vi "Main-Nationa-remotel.vi"() -> ()   [LabVIEW 2019]
uses:
  <userlib>/KNR OS 4.0 LabVIEW Toolkit/F710/f710.ctl
  <vilib>/Platform/TimedLoop/XDataNode/timing_clust.ctl
  <vilib>/Platform/TimedLoop/XDataNode/nitl_modes.ctl
  <vilib>/Platform/TimedLoop/XDataNode/wakeup.ctl
  FPGA_subVIs/low level/motor/motor enum.ctl
  ctl/servo act.ctl
  ctl/remote.ctl
  ctl/height.ctl
  <vilib>/platform/TimedLoop/XDataNode/XDataNode.xnode
  <vilib>/Platform/TimedLoop/XDataNode/XDNodeRunTimeDep.lvlib
  FPGA_subVIs/low level/motor/motor.lvlib
  FPGA_subVIs/my FPGA lib.lvlib
panel:
  out "error out":errorcluster
  in  "stop":bool
  out "Numeric":dbl
  out "-x":dbl
  out "F710":T1
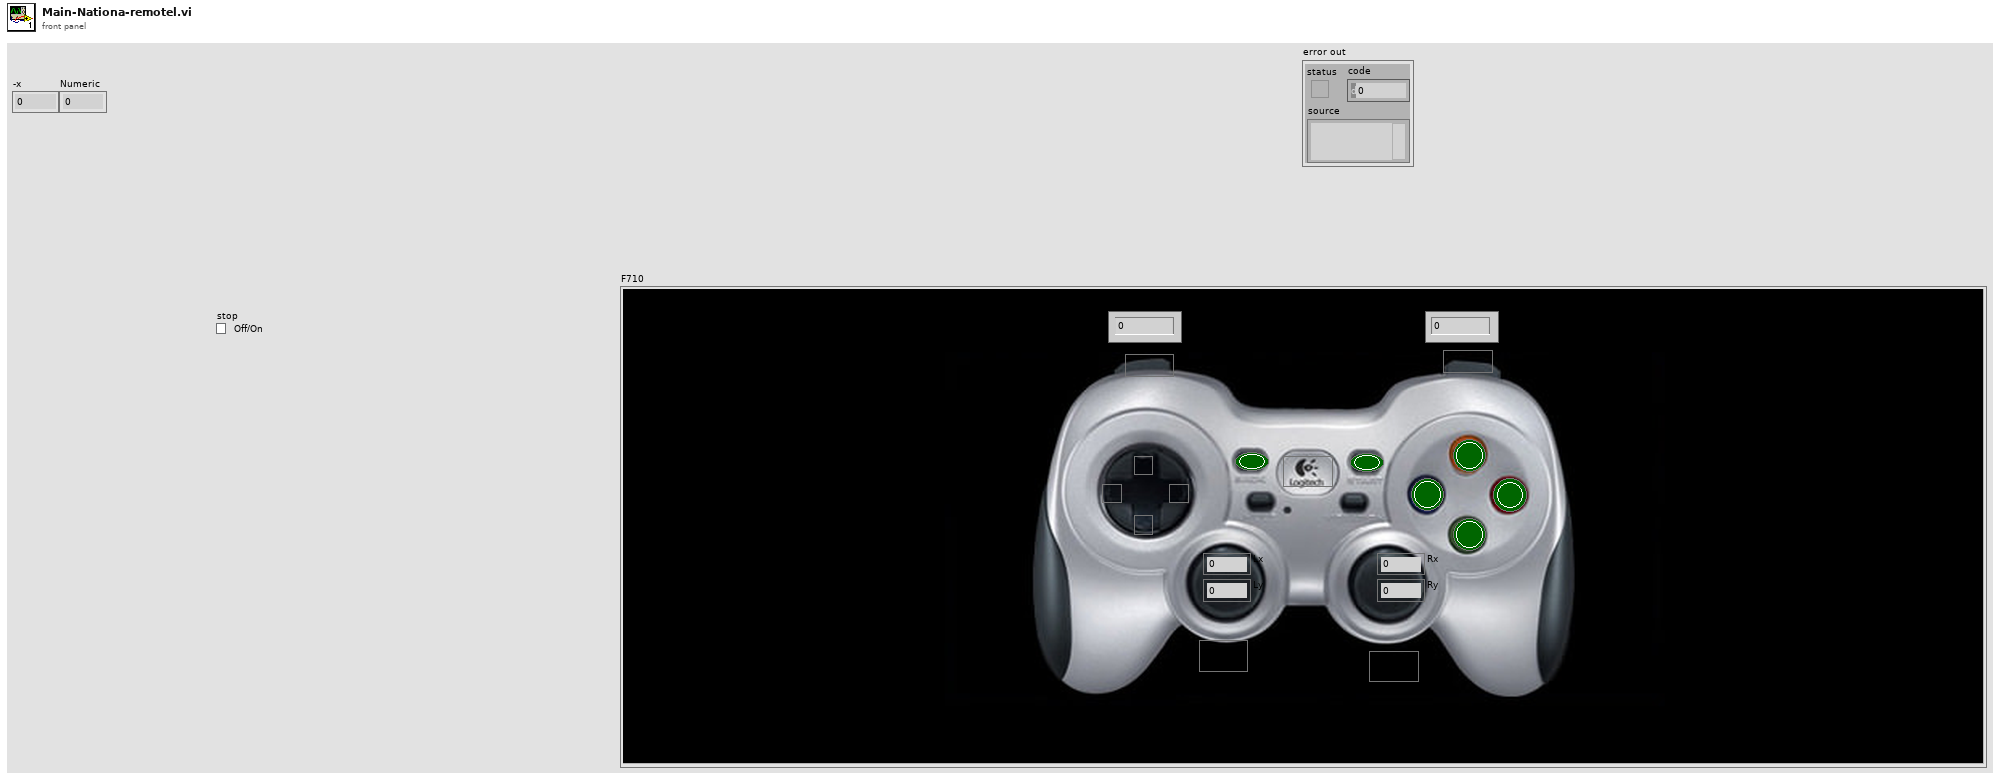
[diagram p1: front panel]
types:
  T1 = typedef "f710.ctl" = cluster{"Down":bool, "Left":bool, "Up":bool, "Right":bool, "A":bool, "X":bool, "Y":bool, "B":bool, "LB":bool, "RB":bool, "LT":i16, "RT":i16, "L3":bool, "R3":bool, "Ly":i16, "Lx":i16, "Ry":i16, "Rx":i16, "Back":bool, "Start":bool, "center":bool}
  T2 = typedef "XDNodeRunTimeDep.lvlib/timing_clust.ctl" = cluster{"Expected End [f-1]":u64, "Actual End [f-1]":u64, "Finished Late? [f-1]":bool, "Expected End [i-1]":u64, "Actual End [i-1]":u64, "Finished Late? [i-1]":bool, "Expected Start [i]":u64, "Actual Start [i]":u64, "Expected Start [f]":u64, "Actual Start [f]":u64, "Source Name":string, "Structure Name":string, "Period":i64, "Deadline":i64, "Offset":i64, "Start":i64, "Priority":i32, "Timeout":i32, "Mode":T3, "Wakeup Reason":T4, "Error":errorcluster, "Source Type":string, "Secondary Source Type":string, "Global End Time":u64, "Global Start Time":u64, "Frame Duration":u64, "Iteration Duration":u64, "Assigned CPU":i32, "I/O Scan Engine Mode":u32}
  T3 = typedef "XDNodeRunTimeDep.lvlib/nitl_modes.ctl" = enum32{"No Change", "Process missed periods, maintain original phase", "Discard missed periods, maintain original phase", "Process missed periods, ignore original phase", "Discard missed periods, ignore original phase"}
  T4 = typedef "XDNodeRunTimeDep.lvlib/wakeup.ctl" = enum32{"Normal", "Aborted", "Asynchronous wakeup", "Timing source error", "Timed loop error", "Timeout"}
  T5 = typedef "servo act.ctl" = enum16{"catch", "relax", "left idle", "center", "red relax", "left reg", "right reg"}
  T6 = cluster{"proportional gain (Kc)":dbl, "integral time (Ti, min)":dbl, "derivative time (Td, min)":dbl}
  T7 = typedef "my FPGA lib.lvlib/motor.lvlib/motor enum.ctl" = enum16{"M1", "M2", "M3", "M4"}
  T8 = typedef "remote.ctl" = cluster{"Motor speed":dbl[], "height":dbl, "dir":i32, "catch?":bool}
  T9 = typedef "height.ctl" = enum16{"IDLE", "recycle pre-catch", "recycle catch", "recycle zone", "vision height", "box 1", "box 2", "box 3", "box 1 pre", "box 2 pre", "box 3 pre", "reg 1", "reg 2", "reg 1 pre", "reg 2 pre", "put 1", "put 2", "put 3"}
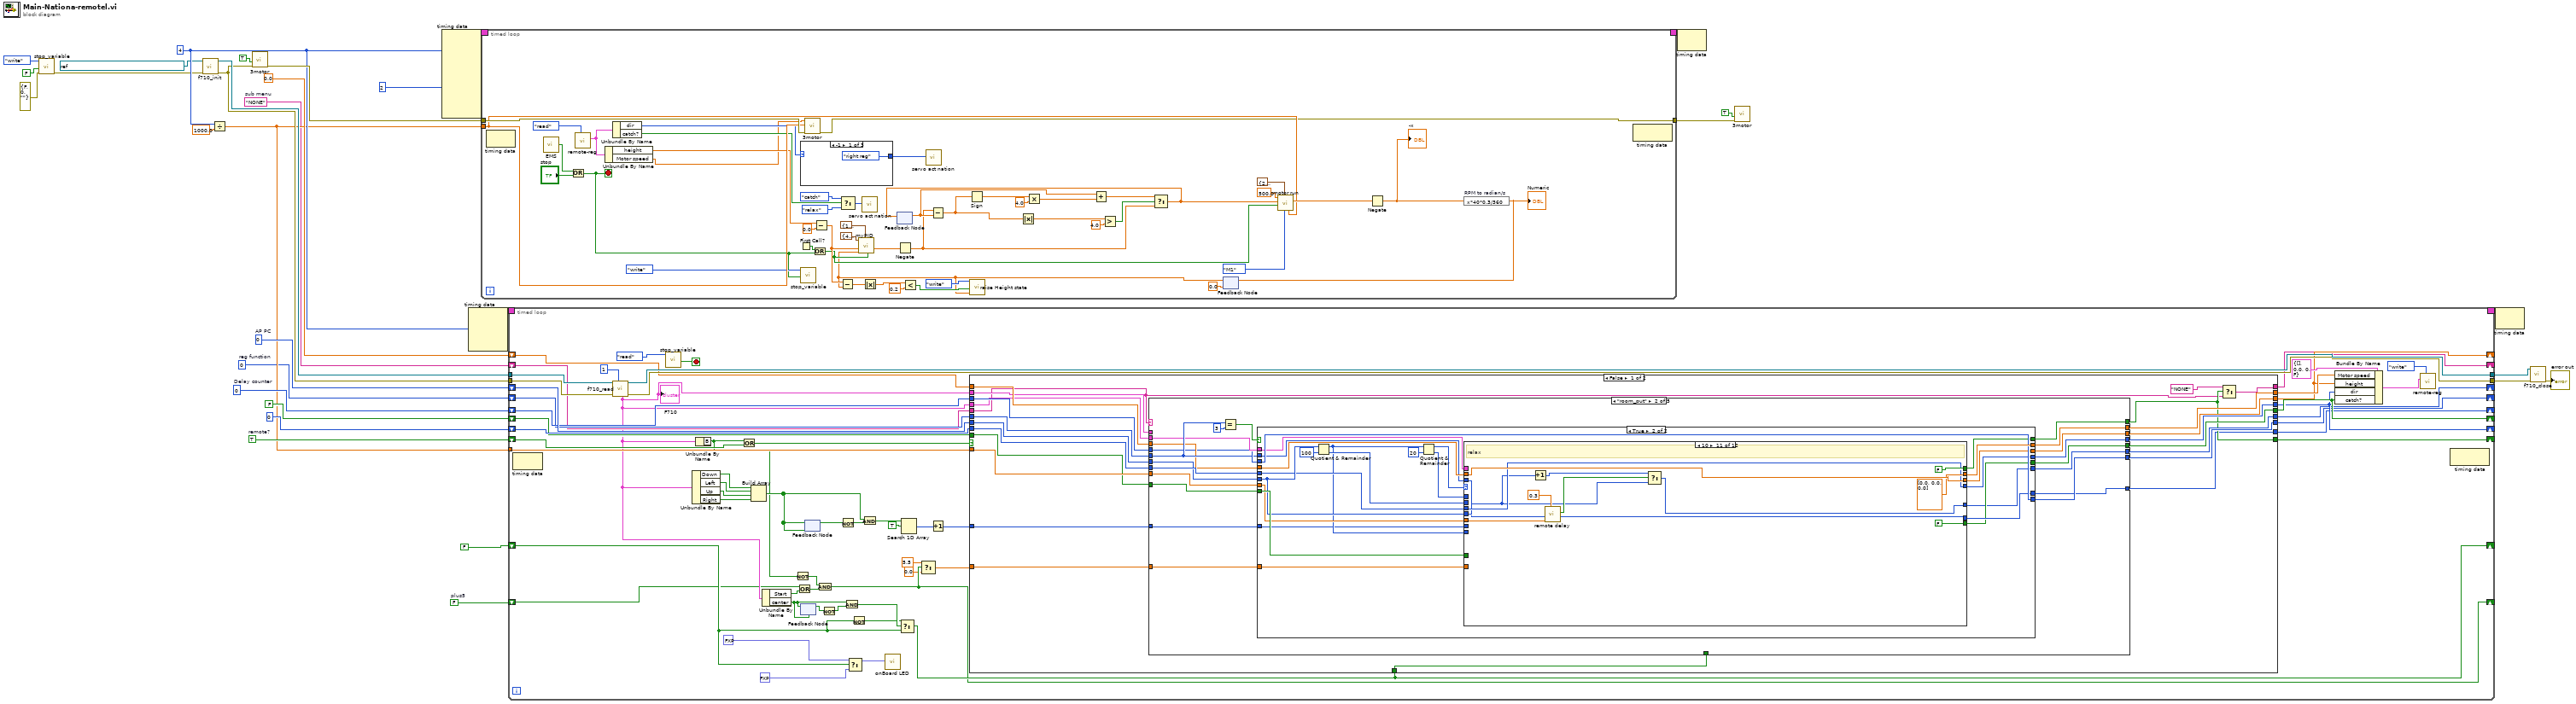
[diagram p0: block diagram]
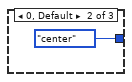
[diagram p2: hidden frame]
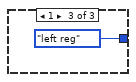
[diagram p3: hidden frame]
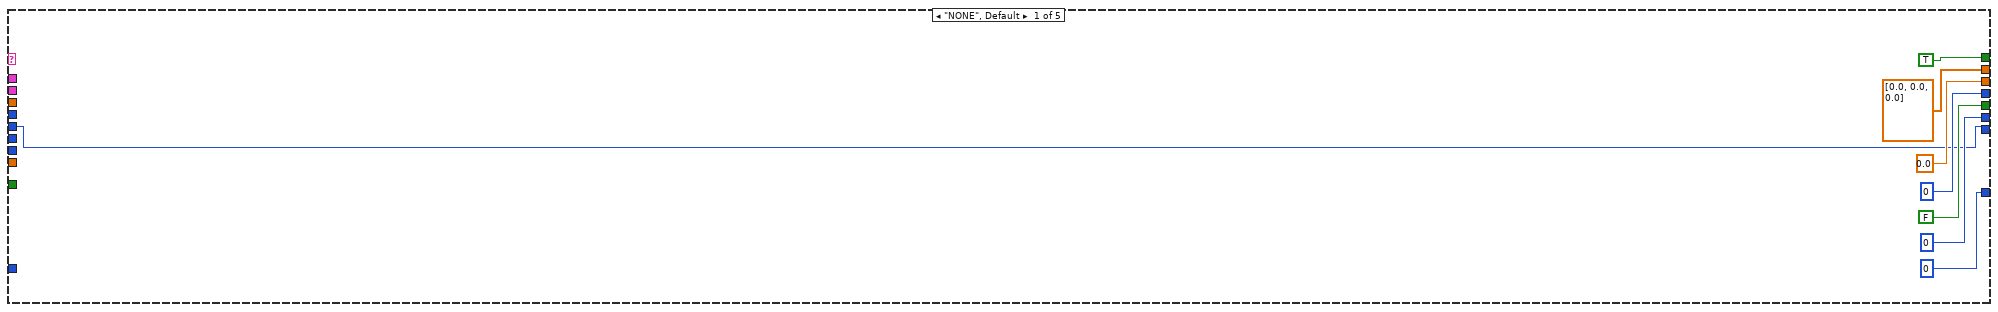
[diagram p4: hidden frame]
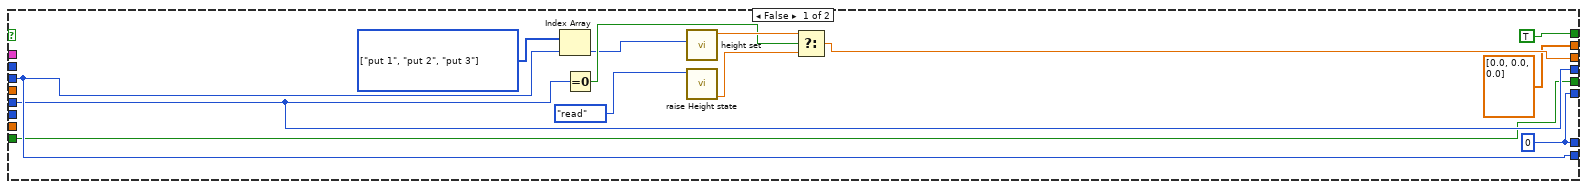
[diagram p5: hidden frame]
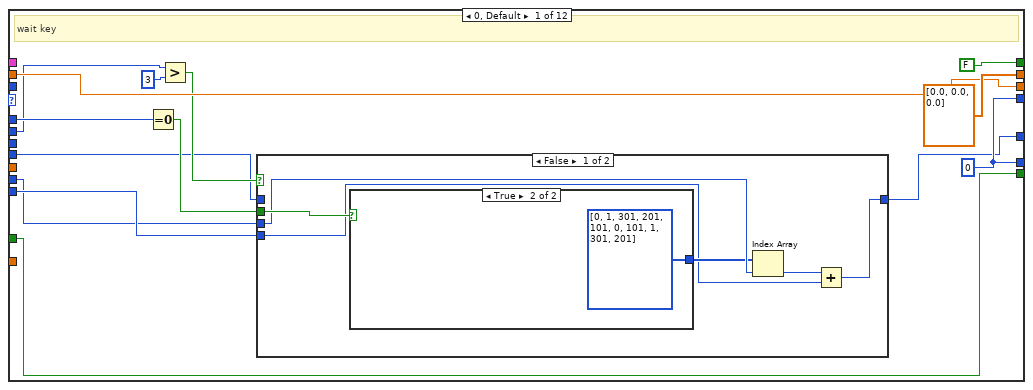
[diagram p6: hidden frame]
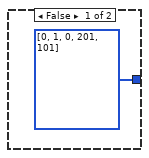
[diagram p7: hidden frame]
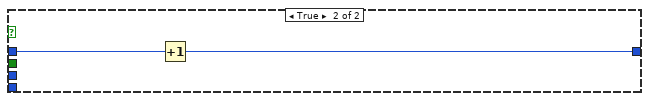
[diagram p8: hidden frame]
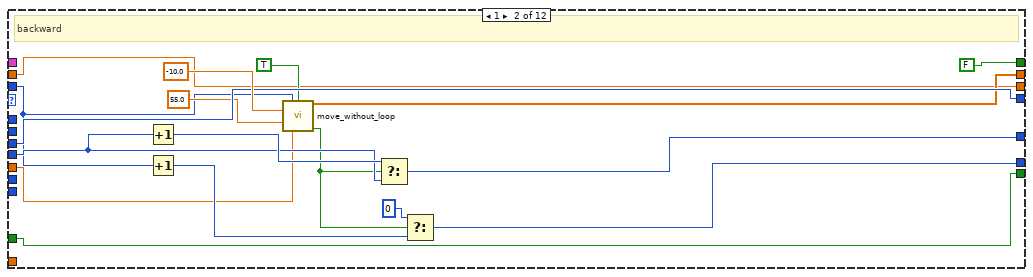
[diagram p9: hidden frame]
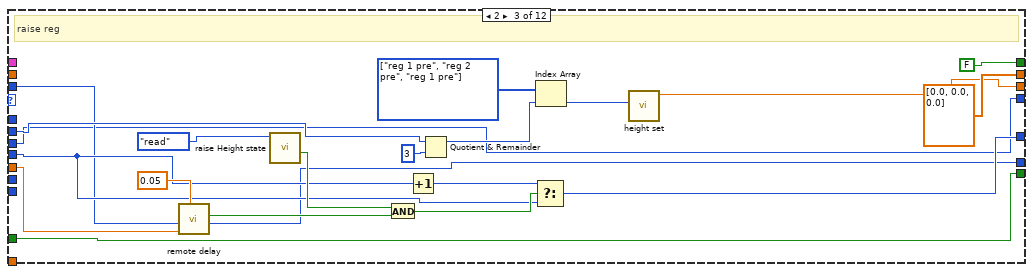
[diagram p10: hidden frame]
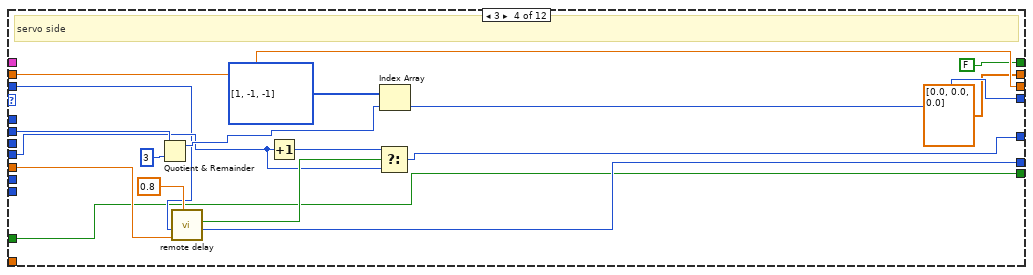
[diagram p11: hidden frame]
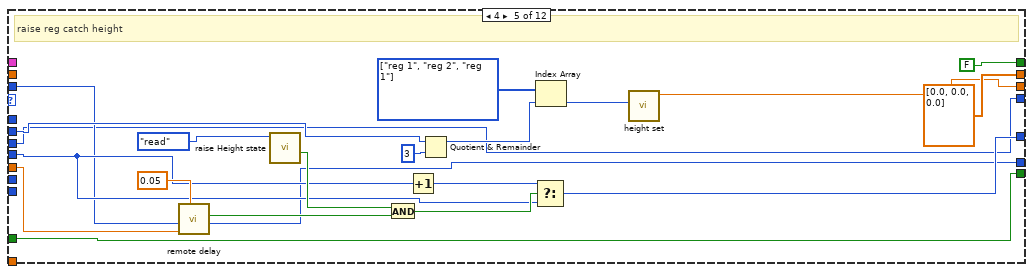
[diagram p12: hidden frame]
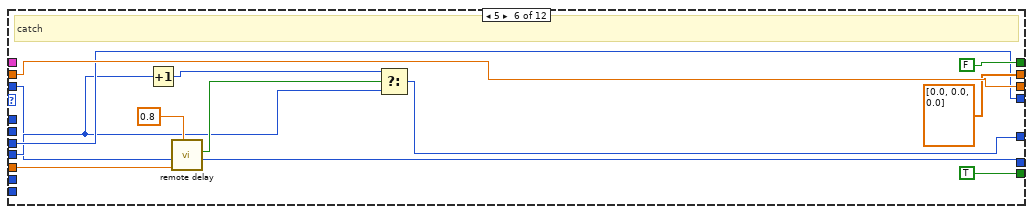
[diagram p13: hidden frame]
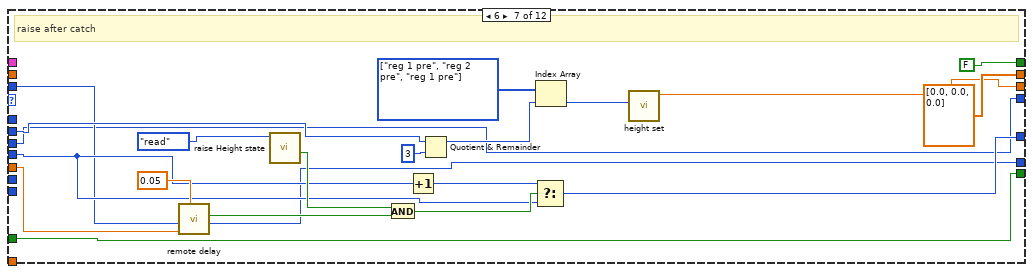
[diagram p14: hidden frame]
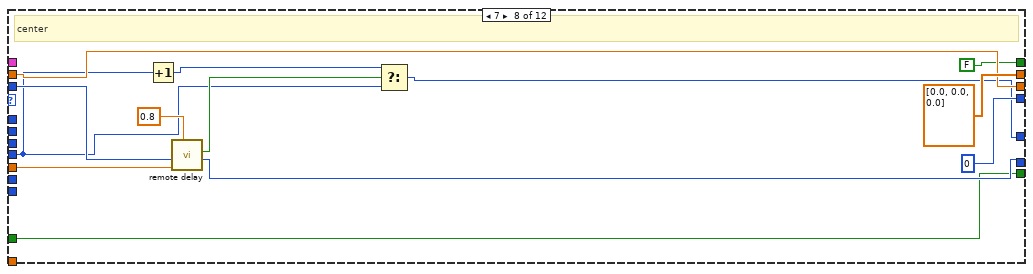
[diagram p15: hidden frame]
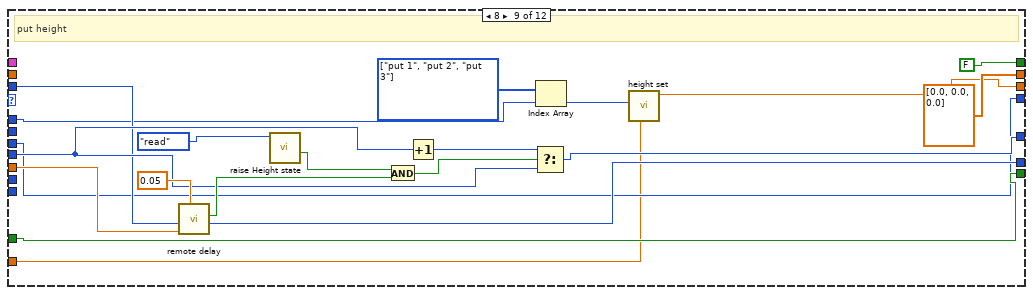
[diagram p16: hidden frame]
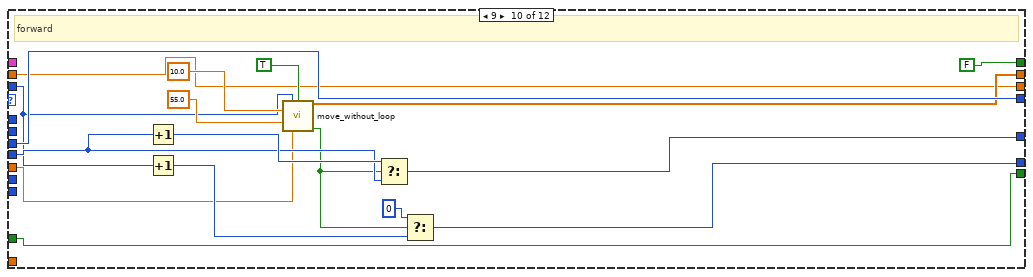
[diagram p17: hidden frame]
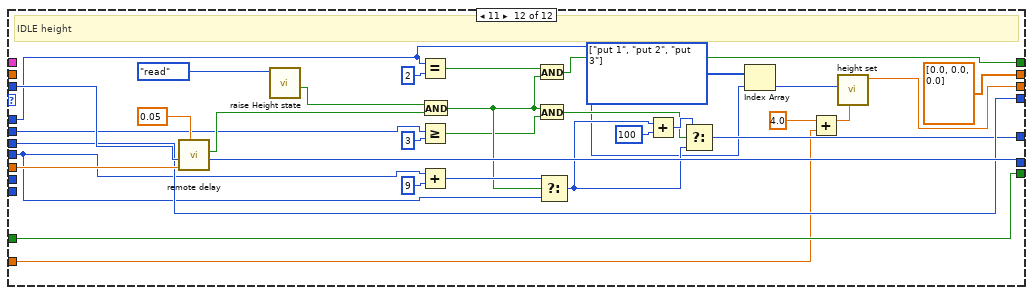
[diagram p18: hidden frame]
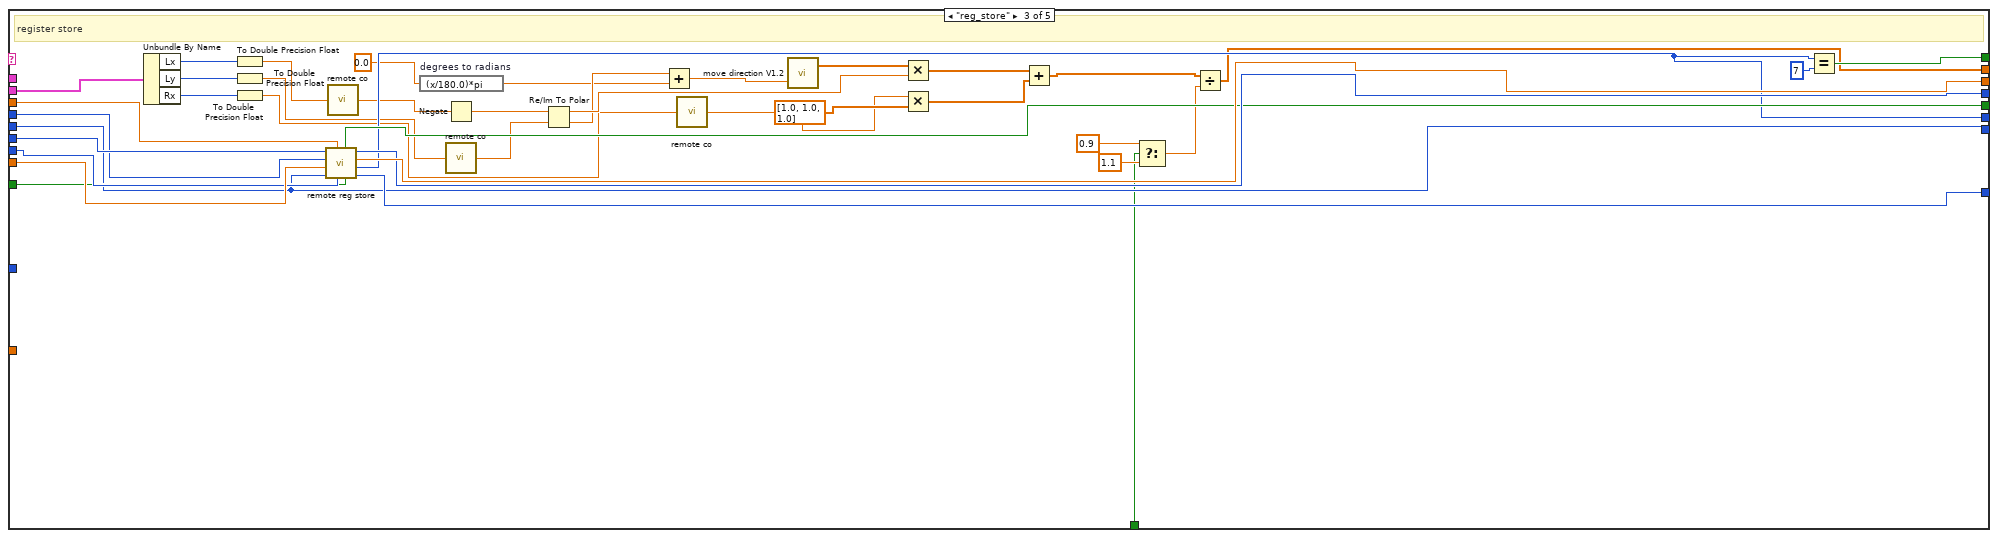
[diagram p19: hidden frame]
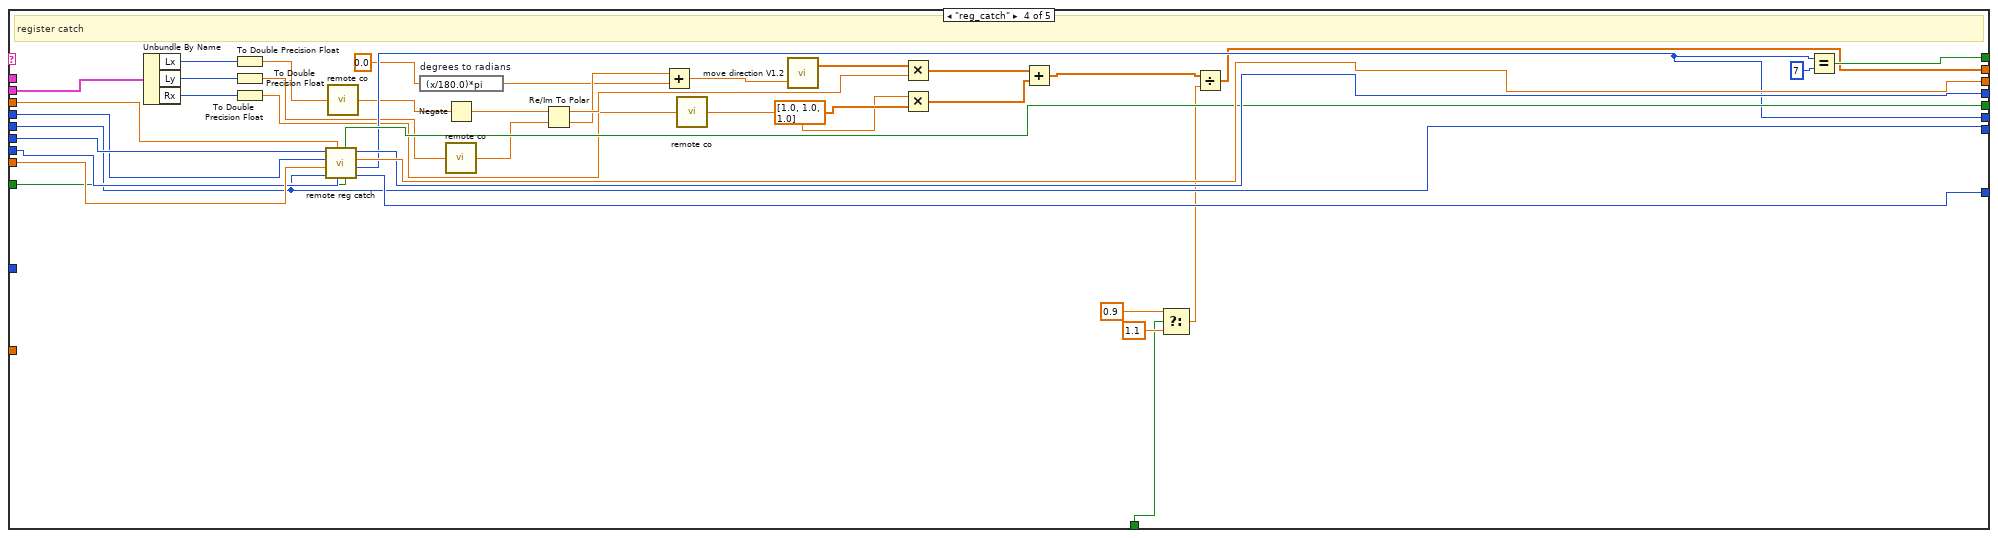
[diagram p20: hidden frame]
diagram:
  w1 = FALSE  # plus5
  w3 = "NONE"  # sub menu
  w4 = 0  # reg function
  w6 = 0  # Delay counter
  w7 = 0  # AP PC
  w8 = TRUE  # remote?
  w23 = i64 4 ("Period")
  n1 = call "stop_variable.vi"("Error In"=errorcluster {"status"=FALSE, "code"=0, "source"=""} ("error in (no error)"), "Write"=FALSE, "Enum"=enum16{"read", "write"}."write") -> ("Error Out"=w12:errorcluster)  [unwired: 7 in, 1 out]
  n2 = call <userlib>:"f710_init.vi"("error in (no error)"=w12, "USB RAW VISA resource name"=refnum<visa-resource-name> "USB0::0x046D::0xC21F::EEAB948F::RAW") -> ("error out"=w11:errorcluster, "VISA Refnum out"=w30:refnum<visa-resource-name>)  [unwired: 8 in]
  n3 = Divide(x=w23, y=1000.0) -> (x/y=w5:dbl)
  n4 = call "3motor.vi"("error in (no error)"=w11, "Reset"=TRUE) -> ("error out"=w25:errorcluster)  [unwired: 8 in, 1 out]
  n5 = node-c288(w23, i64 2 ("Offset")) -> (w27:T2)  [unwired: 8 in]
  n6 = node-c288(w23) -> (w32:T2)  [unwired: 3 in]
  n7 = timed-loop {
    timing: w27 -> [_]
    timing-out: [_] -> w26
    tunnel: w25 -> [w80]
    tunnel: w5 -> [w46]
    tunnel: [w36] -> w21
    stop <- w34 stop-if-true
    n8 = node-c288() -> ()  [unwired: 1 in, 1 out]
    n9 = call "EMS.vi"() -> ("A/DIO4 (Pin 19)"=w61:bool)
    n10 = Or(x=w61, y="stop") -> (x .or. y?=w34:bool)
    n11 = call "remote-reg.vi"("Enum"=enum16{"read", "write"}."read") -> ("read"=w43:T8)  [unwired: 10 in]
    n12 = Unbundle By Name(w43) -> ("height"=w44:dbl, "Motor speed"=w33:dbl[])
    n13 = Unbundle By Name(w43) -> ("dir"=w38:i32, "catch?"=w42:bool)
    n14 = First Call?() -> (First Call?: T/F=w51:bool)
    n15 = case shown="-1" w38 {
      tunnel: [servo_act."right reg" ("servo act") servo_act."center" ("servo act") servo_act."left reg" ("servo act")] -> w37
      frame -1 {
      }
      frame 0, Default {
      }
      frame 1 {
      }
    }
    n16 = call "stop_variable.vi"("Write"=w34, "Enum"=enum16{"read", "write"}."write") -> ()  [unwired: 8 in, 2 out]
    n17 = call "3motor.vi"("error in (no error)"=w80, "dt(s)"=w46, "Motor speed"=w33) -> ("error out"=w36:errorcluster)  [unwired: 7 in, 1 out]
    n18 = Or(x=w51, y=w34) -> (x .or. y?=w48:bool)
    n19 = Subtract(x=w44, y=0.0 ("x")) -> (x-y=w60:dbl)
    n20 = Select(t=servo_act."catch" ("servo act"), s=w42, f=servo_act."relax" ("servo act")) -> (s? t:f=w39:T5)
    n21 = call "servo act nation.vi"("servo act"=w39) -> ()  [unwired: 10 in, 1 out]
    n22 = feedback #1() -> (w71:dbl)  [unwired: 1 in]
    n23 = call "servo act nation.vi"("servo act"=w37) -> ()  [unwired: 10 in, 1 out]
    n24 = feedback #2(0.0) -> (w47:dbl)
    n25 = Subtract(x=w60, y=w47) -> (x-y=w59:dbl)
    n26 = call "myPID.vi"("s"=w48, "output range"=cluster{"output high":dbl, "output low":dbl} {"output high"=140.0, "output low"=-140.0}, "Processer"=w47, "setpoint"=w60, "PID"=cluster{"Kp":dbl, "Ki":dbl, "Kd":dbl} {"Kp"=45.0, "Ki"=0.0, "Kd"=0.0002}) -> ("out"=w75:dbl)  [unwired: 5 in, 1 out]
    n27 = Absolute Value(x=w59) -> (abs(x)=w58:dbl)
    n28 = Negate(x=w75) -> (-x=w66:dbl)
    n29 = Less?(x=w58, y=0.2) -> (x < y?=w56:bool)
    n30 = Subtract(x=w66, y=w71) -> (x-y=w65:dbl)
    n31 = Sign(1:w65) -> (0:w70:dbl)
    n32 = call "raise Height state.vi"("Write Height"=w47, "Write"=w56, "Enum"=enum16{"read", "write"}."write") -> ()  [unwired: 7 in, 2 out]
    n33 = Absolute Value(x=w65) -> (abs(x)=w74:dbl)
    n34 = Multiply(x=w70, y=4.0) -> (x*y=w68:dbl)
    n35 = Add(x=w71, y=w68) -> (x+y=w67:dbl)
    n36 = Greater?(x=w74, y=4.0) -> (0:w72:bool)
    n37 = Select(t=w67, s=w72, f=w66) -> (s? t:f=w53:dbl)
    n38 = feedback-in #1(w53) -> ()
    n39 = call "motor run.vi"("dt(s)"=w46, "motor select"=motor_enum."M1", "PID gains"=T6 {"proportional gain (Kc)"=20.0, "integral time (Ti, min)"=0.0, "derivative time (Td, min)"=0.0002}, "Reset"=w48, "speed RPM"=w53, "PWM frequence"=500.0) -> ("encoder"=w49:dbl)  [unwired: 2 in, 3 out]
    n40 = Negate(x=w49) -> (-x=w76:dbl)
    "-x" <- w76
    n41 = expression code="x*40*0.3/360" "RPM to radian/s"(w76) -> (w63:dbl)
    "Numeric" <- w63
    n42 = feedback-in #2(w63) -> ()
    n43 = node-c288() -> ()  [unwired: 1 in, 1 out]
  }
  n44 = timed-loop {
    timing: w32 -> [_]
    timing-out: [_] -> w31
    tunnel: w11 -> [w145]
    tunnel: w30 -> [w144]
    tunnel: [w143] -> w29
    tunnel: [w142] -> w28
    shift-right: [w129] -> _
    shift-left: 0.0 -> [w136]
    shift-right: [w128] -> _
    shift-left: 0 -> [w133]
    shift-right: [w130] -> _
    shift-left: FALSE -> [w132]
    shift-right: [w127] -> _
    shift-left: w8 -> [w131]
    shift-right: [w125] -> _
    shift-left: w7 -> [w126]
    shift-right: [w123] -> _
    shift-left: w6 -> [w124]
    tunnel: w5 -> [w122]
    shift-right: [w120] -> _
    shift-left: w4 -> [w121]
    shift-right: [w117] -> _
    shift-left: w3 -> [w118]
    shift-right: [w99] -> _
    shift-left: FALSE -> [w96]
    shift-right: [w89] -> _
    shift-left: w1 -> [w94]
    stop <- w140 stop-if-true
    n45 = node-c288() -> ()  [unwired: 1 in, 1 out]
    n46 = call <userlib>:"f710_read.vi"("Timeout to wait for Interrupt (ms)"=u32 1, "error in (no error)"=w145, "VISA Refnum in"=w144) -> ("error out"=w142:errorcluster, "VISA Refnum out"=w143:refnum<visa-resource-name>, "F710"=w102:T1)  [unwired: 6 in]
    "F710" <- w102
    n47 = call "stop_variable.vi"("Enum"=enum16{"read", "write"}."read") -> ("read"=w140:bool)  [unwired: 9 in, 1 out]
    n48 = Unbundle By Name(w102) -> ("Down"=w112:bool, "Left"=w113:bool, "Up"=w114:bool, "Right"=w115:bool)
    n49 = Unbundle By Name(w102) -> ("B"=w90:bool)
    n50 = Or(x=w90, y=w131) -> (x .or. y?=w119:bool)
    n51 = Build Array(w112, w113, w114, w115) -> (w109:bool[])
    n52 = Unbundle By Name(w102) -> ("Start"=w93:bool, "center"=w105:bool)
    n53 = Not(x=w90) -> (.not. x?=w91:bool)
    n54 = Or(x=w94, y=w93) -> (x .or. y?=w92:bool)
    n55 = feedback #3(w105) -> (w103:bool)
    n56 = feedback-in #3(w105) -> ()
    n57 = feedback #4(w109) -> (w108:bool[])
    n58 = feedback-in #4(w109) -> ()
    n59 = And(x=w91, y=w92) -> (x .and. y?=w89:bool)
    n60 = Not(x=w103) -> (.not. x?=w104:bool)
    n61 = Not(x=w108) -> (.not. x?=w110:bool[])
    n62 = And(x=w105, y=w104) -> (x .and. y?=w101:bool)
    n63 = Select(t=fxp<+,4,4> 15.0 ("OnBoard.LED[3:0]"), s=w96, f=fxp<+,4,4> 0.0 ("OnBoard.LED[3:0]")) -> (s? t:f=w97:fxp<+,4,4>)
    n64 = Not(x=w96) -> (.not. x?=w100:bool)
    n65 = And(x=w109, y=w110) -> (x .and. y?=w111:bool[])
    n66 = call "onBoard LED.vi"("OnBoard.LED[3:0]"=w97) -> ()  [unwired: 10 in, 1 out]
    n67 = Select(t=w100, s=w101, f=w96) -> (s? t:f=w99:bool)
    n68 = Search 1D Array(1D array=w111, element=TRUE) -> (index of element=w116:i32)  [unwired: 1 in]
    n69 = Select(t=5.5, s=w89, f=0.0) -> (s? t:f=w86:dbl)
    n70 = Increment(x=w116) -> (x+1=w106:i32)
    n71 = case shown="False" w119 {
      selector: w119 -> [_ w591]
      tunnel: [w168 w630] -> w137
      tunnel: w136 -> [w164 w623]
      tunnel: [w165 w569] -> w129
      tunnel: w102 -> [w157 w559]
      tunnel: w133 -> [w160 w613]
      tunnel: [w162 w593] -> w128
      tunnel: w132 -> [w159 w596]
      tunnel: [w158 w595] -> w130
      tunnel: [w153 w592] -> w127
      tunnel: w126 -> [w167 _]
      tunnel: [w163 w589] -> w125
      tunnel: w124 -> [w166 _]
      tunnel: [w149 w589] -> w123
      tunnel: w122 -> [w161 _]
      tunnel: w102 -> [w156 _]
      tunnel: w121 -> [w155 _]
      tunnel: [w154 w574] -> w120
      tunnel: w118 -> [w152 w571]
      tunnel: [w150 w576] -> w117
      tunnel: w106 -> [w148 _]
      tunnel: w99 -> [w147 w557]
      tunnel: w86 -> [w146 _]
      frame False {
        n72 = case shown="\"room_put\"" w152 {
          tunnel: [dbl[] [0.0, 0.0, 0.0] w184 w466 w506 dbl[] [0.0, 0.0, 0.0]] -> w168
          tunnel: w167 -> [_ w183 w501 w541 _]
          tunnel: w166 -> [_ w180 w500 w540 _]
          tunnel: [0.0 ("upper limit") w190 w499 w539 w546] -> w165
          tunnel: w164 -> [_ w182 w498 w538 _]
          tunnel: [0 ("Delay counter") w187 w497 w537 0 ("delay timer out")] -> w149
          tunnel: [0 w188 w490 w530 0 ("PC out")] -> w163
          tunnel: [0 w191 w496 w536 w550] -> w162
          tunnel: w161 -> [_ w179 w495 w535 _]
          tunnel: w160 -> [_ w192 w494 w534 w550]
          tunnel: w159 -> [_ w185 w493 w533 w553]
          tunnel: [FALSE w186 w492 w532 w553] -> w158
          tunnel: [TRUE w189 w491 w531 TRUE] -> w153
          tunnel: w157 -> [_ w181 w467 w507 _]
          tunnel: w156 -> [_ _ _ _ _]
          tunnel: w155 -> [w169 w194 w488 w528 w542]
          tunnel: [w169 w193 w488 w528 w542] -> w154
          tunnel: w148 -> [_ w178 _ _ _]
          tunnel: w147 -> [_ _ w462 w503 _]
          tunnel: w146 -> [_ w177 _ _ _]
          frame "NONE", Default {
          }
          frame "room_put" {
            n73 = Equal?(x=w194, y=3) -> (x = y?=w195:bool)
            n74 = case shown="True" w195 {
              tunnel: w194 -> [w203 w231]
              tunnel: [w203 w231] -> w193
              tunnel: w192 -> [w202 w215]
              tunnel: [w202 w230] -> w191
              tunnel: [w201 w225] -> w190
              tunnel: [TRUE w228] -> w189
              tunnel: [w199 w216] -> w188
              tunnel: [w199 w229] -> w187
              tunnel: [w198 w227] -> w186
              tunnel: w185 -> [w198 w226]
              tunnel: [dbl[] [0.0, 0.0, 0.0] w232] -> w184
              tunnel: w183 -> [_ w217]
              tunnel: w182 -> [_ w224]
              tunnel: w181 -> [_ w223]
              tunnel: w180 -> [_ w214]
              tunnel: w179 -> [_ w213]
              tunnel: w178 -> [_ w211]
              tunnel: w177 -> [_ w210]
              frame False {
                w199 = 0
                w205 = T9[] [enum."put 1", enum."put 2", enum."put 3"] items=["IDLE", "recycle pre-catch", "recycle catch", "recycle zone", "vision height", "box 1", "box 2", "box 3", "box 1 pre", "box 2 pre", "box 3 pre", "reg 1", "reg 2", "reg 1 pre", "reg 2 pre", "put 1", "put 2", "put 3"] ("height name")
                n75 = Index Array(array=w205, index=w203) -> (element=w204:T9)
                n76 = Equal To 0?(x=w202) -> (x = 0?=w208:bool)
                n77 = call "height set.vi"("height name"=w204) -> ("Numeric"=w209:dbl)  [unwired: 10 in]
                n78 = call "raise Height state.vi"("Enum"=enum16{"read", "write"}."read") -> ("read Height"=w206:dbl)  [unwired: 9 in, 1 out]
                n79 = Select(t=w209, s=w208, f=w206) -> (s? t:f=w201:dbl)
              }
              frame True {
                n80 = Quotient & Remainder(x=w217, y=100) -> (x-y*floor(x/y)=w212:i32, floor(x/y)=w218:i32)
                n81 = Quotient & Remainder(x=w212, y=20) -> (x-y*floor(x/y)=w221:i32, floor(x/y)=w220:i32)
                n82 = case shown="10" w221 {
                  tunnel: [dbl[] [0.0, 0.0, 0.0] w260 dbl[] [0.0, 0.0, 0.0] dbl[] [0.0, 0.0, 0.0] dbl[] [0.0, 0.0, 0.0] dbl[] [0.0, 0.0, 0.0] dbl[] [0.0, 0.0, 0.0] dbl[] [0.0, 0.0, 0.0] dbl[] [0.0, 0.0, 0.0] w403 dbl[] [0.0, 0.0, 0.0] dbl[] [0.0, 0.0, 0.0]] -> w232
                  tunnel: [w245 w272 w274 w307 w312 w341 w346 0 ("Numeric") w382 w415 w425 w452] -> w230
                  tunnel: [w245 w267 w278 w298 w316 w336 w350 w373 w386 w410 w420 w456] -> w229
                  tunnel: [FALSE FALSE FALSE FALSE FALSE FALSE FALSE FALSE FALSE FALSE FALSE w446] -> w228
                  tunnel: [w243 w258 w275 w295 w313 TRUE w347 w367 w383 w401 FALSE w453] -> w227
                  tunnel: w226 -> [w243 w258 w275 w295 w313 _ w347 w367 w383 w401 _ w453]
                  tunnel: [w242 w257 w288 w306 w326 w343 w360 w377 w396 w400 w427 w434] -> w225
                  tunnel: w224 -> [w242 w257 _ w306 _ w343 _ w377 _ w400 w427 _]
                  tunnel: w223 -> [_ _ _ _ _ _ _ _ _ _ _ _]
                  tunnel: w220 -> [w241 _ _ _ _ _ _ _ w381 _ _ w432]
                  tunnel: w218 -> [w239 _ w294 w310 w332 _ w366 _ _ _ _ w444]
                  tunnel: w217 -> [w236 w269 w279 w299 w317 w337 w351 w370 w387 w412 w421 w450]
                  tunnel: [w235 w271 w280 w300 w318 w335 w352 w369 w388 w414 w419 w445] -> w216
                  tunnel: w215 -> [_ w272 w274 _ w312 w341 w346 _ w382 w415 w425 w452]
                  tunnel: w214 -> [_ w262 w277 w297 w315 w334 w349 w372 w385 w405 w418 w455]
                  tunnel: w213 -> [_ w264 w276 w296 w314 w333 w348 w371 w384 w407 w417 w454]
                  tunnel: w212 -> [w234 _ _ _ _ _ _ _ _ _ _ _]
                  tunnel: w211 -> [w233 _ _ _ _ _ _ _ _ _ _ _]
                  tunnel: w210 -> [_ _ _ _ _ _ _ _ w380 _ _ w430]
                  frame 0, Default {
                    w245 = 0
                    # "wait key"
                    n83 = Equal To 0?(x=w241) -> (x = 0?=w240:bool)
                    n84 = Greater?(x=w239, y=3) -> (0:w237:bool)
                    n85 = case shown="False" w237 {
                      tunnel: w240 -> [w252 _]
                      tunnel: w233 -> [w251 _]
                      tunnel: w236 -> [_ w256]
                      tunnel: [w248 w255] -> w235
                      tunnel: w234 -> [w247 _]
                      frame False {
                        n86 = case shown="True" w252 {
                          tunnel: [i32[] [0, 1, 0, 201, 101] i32[] [0, 1, 301, 201, 101, 0, 101, 1, 301, 201]] -> w250
                          frame False {
                          }
                          frame True {
                          }
                        }
                        n87 = Index Array(array=w250, index=w251) -> (element=w249:i32)
                        n88 = Add(x=w249, y=w247) -> (x+y=w248:i32)
                      }
                      frame True {
                        n89 = Increment(x=w256) -> (x+1=w255:i32)
                      }
                    }
                  }
                  frame 1 {
                    # "backward"
                    n90 = Increment(x=w269) -> (x+1=w270:i32)
                    n91 = Increment(x=w262) -> (x+1=w268:i32)
                    n92 = call "move_without_loop.vi"("i"=w262, "run"=TRUE, "Y"=-10.0, "speed"=55.0, "dt"=w264) -> ("speed out"=w260:dbl[], "complet"=w266:bool)  [unwired: 6 in, 3 out]
                    n93 = Select(t=w270, s=w266, f=w269) -> (s? t:f=w271:i32)
                    n94 = Select(t=0, s=w266, f=w268) -> (s? t:f=w267:i32)
                  }
                  frame 2 {
                    w292 = T9[] [enum."reg 1 pre", enum."reg 2 pre", enum."reg 1 pre"] items=["IDLE", "recycle pre-catch", "recycle catch", "recycle zone", "vision height", "box 1", "box 2", "box 3", "box 1 pre", "box 2 pre", "box 3 pre", "reg 1", "reg 2", "reg 1 pre", "reg 2 pre", "put 1", "put 2", "put 3"] ("height name")
                    # "raise reg"
                    n95 = call "remote delay.vi"("second"=0.05, "dt(s)"=w276, "i"=w277) -> ("i out"=w278:i32, "finish?"=w282:bool)  [unwired: 7 in]
                    n96 = call "raise Height state.vi"("Enum"=enum16{"read", "write"}."read") -> ("read"=w283:bool)  [unwired: 9 in, 1 out]
                    n97 = And(x=w283, y=w282) -> (x .and. y?=w281:bool)
                    n98 = Increment(x=w279) -> (x+1=w285:i32)
                    n99 = Quotient & Remainder(x=w294, y=3) -> (x-y*floor(x/y)=w289:i32)  [unwired: 1 out]
                    n100 = Select(t=w285, s=w281, f=w279) -> (s? t:f=w280:i32)
                    n101 = Index Array(array=w292, index=w289) -> (element=w291:T9)
                    n102 = call "height set.vi"("height name"=w291) -> ("Numeric"=w288:dbl)  [unwired: 10 in]
                  }
                  frame 3 {
                    # "servo side"
                    n103 = Quotient & Remainder(x=w310, y=3) -> (x-y*floor(x/y)=w308:i32)  [unwired: 1 out]
                    n104 = call "remote delay.vi"("second"=0.8, "dt(s)"=w296, "i"=w297) -> ("i out"=w298:i32, "finish?"=w302:bool)  [unwired: 7 in]
                    n105 = Increment(x=w299) -> (x+1=w301:i32)
                    n106 = Select(t=w301, s=w302, f=w299) -> (s? t:f=w300:i32)
                    n107 = Index Array(array=i32[] [1, -1, -1], index=w308) -> (element=w307:i32)
                  }
                  frame 4 {
                    w330 = T9[] [enum."reg 1", enum."reg 2", enum."reg 1"] items=["IDLE", "recycle pre-catch", "recycle catch", "recycle zone", "vision height", "box 1", "box 2", "box 3", "box 1 pre", "box 2 pre", "box 3 pre", "reg 1", "reg 2", "reg 1 pre", "reg 2 pre", "put 1", "put 2", "put 3"] ("height name")
                    # "raise reg catch height"
                    n108 = call "remote delay.vi"("second"=0.05, "dt(s)"=w314, "i"=w315) -> ("i out"=w316:i32, "finish?"=w320:bool)  [unwired: 7 in]
                    n109 = call "raise Height state.vi"("Enum"=enum16{"read", "write"}."read") -> ("read"=w321:bool)  [unwired: 9 in, 1 out]
                    n110 = And(x=w321, y=w320) -> (x .and. y?=w319:bool)
                    n111 = Increment(x=w317) -> (x+1=w323:i32)
                    n112 = Quotient & Remainder(x=w332, y=3) -> (x-y*floor(x/y)=w327:i32)  [unwired: 1 out]
                    n113 = Select(t=w323, s=w319, f=w317) -> (s? t:f=w318:i32)
                    n114 = Index Array(array=w330, index=w327) -> (element=w329:T9)
                    n115 = call "height set.vi"("height name"=w329) -> ("Numeric"=w326:dbl)  [unwired: 10 in]
                  }
                  frame 5 {
                    # "catch"
                    n116 = Increment(x=w337) -> (x+1=w338:i32)
                    n117 = call "remote delay.vi"("second"=0.8, "dt(s)"=w333, "i"=w334) -> ("i out"=w336:i32, "finish?"=w339:bool)  [unwired: 7 in]
                    n118 = Select(t=w338, s=w339, f=w337) -> (s? t:f=w335:i32)
                  }
                  frame 6 {
                    w364 = T9[] [enum."reg 1 pre", enum."reg 2 pre", enum."reg 1 pre"] items=["IDLE", "recycle pre-catch", "recycle catch", "recycle zone", "vision height", "box 1", "box 2", "box 3", "box 1 pre", "box 2 pre", "box 3 pre", "reg 1", "reg 2", "reg 1 pre", "reg 2 pre", "put 1", "put 2", "put 3"] ("height name")
                    # "raise after catch"
                    n119 = call "remote delay.vi"("second"=0.05, "dt(s)"=w348, "i"=w349) -> ("i out"=w350:i32, "finish?"=w354:bool)  [unwired: 7 in]
                    n120 = call "raise Height state.vi"("Enum"=enum16{"read", "write"}."read") -> ("read"=w355:bool)  [unwired: 9 in, 1 out]
                    n121 = And(x=w355, y=w354) -> (x .and. y?=w353:bool)
                    n122 = Increment(x=w351) -> (x+1=w357:i32)
                    n123 = Quotient & Remainder(x=w366, y=3) -> (x-y*floor(x/y)=w361:i32)  [unwired: 1 out]
                    n124 = Select(t=w357, s=w353, f=w351) -> (s? t:f=w352:i32)
                    n125 = Index Array(array=w364, index=w361) -> (element=w363:T9)
                    n126 = call "height set.vi"("height name"=w363) -> ("Numeric"=w360:dbl)  [unwired: 10 in]
                  }
                  frame 7 {
                    # "center"
                    n127 = Increment(x=w370) -> (x+1=w374:i32)
                    n128 = call "remote delay.vi"("second"=0.8, "dt(s)"=w371, "i"=w372) -> ("i out"=w373:i32, "finish?"=w375:bool)  [unwired: 7 in]
                    n129 = Select(t=w374, s=w375, f=w370) -> (s? t:f=w369:i32)
                  }
                  frame 8 {
                    w399 = T9[] [enum."put 1", enum."put 2", enum."put 3"] items=["IDLE", "recycle pre-catch", "recycle catch", "recycle zone", "vision height", "box 1", "box 2", "box 3", "box 1 pre", "box 2 pre", "box 3 pre", "reg 1", "reg 2", "reg 1 pre", "reg 2 pre", "put 1", "put 2", "put 3"] ("height name")
                    # "put height"
                    n130 = call "remote delay.vi"("second"=0.05, "dt(s)"=w384, "i"=w385) -> ("i out"=w386:i32, "finish?"=w390:bool)  [unwired: 7 in]
                    n131 = call "raise Height state.vi"("Enum"=enum16{"read", "write"}."read") -> ("read"=w391:bool)  [unwired: 9 in, 1 out]
                    n132 = And(x=w391, y=w390) -> (x .and. y?=w389:bool)
                    n133 = Increment(x=w387) -> (x+1=w393:i32)
                    n134 = Select(t=w393, s=w389, f=w387) -> (s? t:f=w388:i32)
                    n135 = Index Array(array=w399, index=w381) -> (element=w398:T9)
                    n136 = call "height set.vi"("offset"=w380, "height name"=w398) -> ("Numeric"=w396:dbl)  [unwired: 9 in]
                  }
                  frame 9 {
                    # "forward"
                    n137 = Increment(x=w412) -> (x+1=w413:i32)
                    n138 = Increment(x=w405) -> (x+1=w411:i32)
                    n139 = call "move_without_loop.vi"("i"=w405, "run"=TRUE, "Y"=10.0, "speed"=55.0, "dt"=w407) -> ("speed out"=w403:dbl[], "complet"=w409:bool)  [unwired: 6 in, 3 out]
                    n140 = Select(t=w413, s=w409, f=w412) -> (s? t:f=w414:i32)
                    n141 = Select(t=0, s=w409, f=w411) -> (s? t:f=w410:i32)
                  }
                  frame 10 {
                    # "relax"
                    n142 = Increment(x=w421) -> (x+1=w422:i32)
                    n143 = call "remote delay.vi"("second"=0.3, "dt(s)"=w417, "i"=w418) -> ("i out"=w420:i32, "finish?"=w423:bool)  [unwired: 7 in]
                    n144 = Select(t=w422, s=w423, f=w421) -> (s? t:f=w419:i32)
                  }
                  frame 11 {
                    w436 = T9[] [enum."put 1", enum."put 2", enum."put 3"] items=["IDLE", "recycle pre-catch", "recycle catch", "recycle zone", "vision height", "box 1", "box 2", "box 3", "box 1 pre", "box 2 pre", "box 3 pre", "reg 1", "reg 2", "reg 1 pre", "reg 2 pre", "put 1", "put 2", "put 3"] ("height name")
                    # "IDLE height"
                    n145 = call "remote delay.vi"("second"=0.05, "dt(s)"=w454, "i"=w455) -> ("i out"=w456:i32, "finish?"=w457:bool)  [unwired: 7 in]
                    n146 = call "raise Height state.vi"("Enum"=enum16{"read", "write"}."read") -> ("read"=w458:bool)  [unwired: 9 in, 1 out]
                    n147 = Equal?(x=w432, y=2) -> (x = y?=w447:bool)
                    n148 = Greater Or Equal?(x=w444, y=3) -> (x >= y?=w438:bool)
                    n149 = Add(x=w450, y=9) -> (x+y=w451:i32)
                    n150 = And(x=w458, y=w457) -> (x .and. y?=w439:bool)
                    n151 = And(x=w447, y=w439) -> (x .and. y?=w446:bool)
                    n152 = And(x=w439, y=w438) -> (x .and. y?=w437:bool)
                    n153 = Select(t=w451, s=w439, f=w450) -> (s? t:f=w442:i32)
                    n154 = Add(x=w442, y=100) -> (x+y=w441:i32)
                    n155 = Select(t=w441, s=w437, f=w442) -> (s? t:f=w445:i32)
                    n156 = Index Array(array=w436, index=w432) -> (element=w435:T9)
                    n157 = Add(x=4.0 ("offset"), y=w430) -> (x+y=w431:dbl)
                    n158 = call "height set.vi"("offset"=w431, "height name"=w435) -> ("Numeric"=w434:dbl)  [unwired: 9 in]
                  }
                }
              }
            }
          }
          frame "reg_store" {
            # "register store"
            n159 = Unbundle By Name(w467) -> ("Lx"=w487:i16, "Ly"=w486:i16, "Rx"=w485:i16)
            n160 = To Double Precision Float(number=w487) -> (double precision float=w477:dbl)
            n161 = To Double Precision Float(number=w486) -> (double precision float=w475:dbl)
            n162 = To Double Precision Float(number=w485) -> (double precision float=w472:dbl)
            n163 = call "remote reg store.vi"("catch? in"=w493, "dir in"=w494, "height in"=w498, "reg"=w488, "dt"=w495, "delay timer in"=w500, "PC in"=w501) -> ("delay timer out"=w497:i32, "PC out"=w490:i32, "height out"=w499:dbl, "dir out"=w496:i32, "catch? out"=w492:bool)
            n164 = call "remote co.vi"("input"=w477) -> ("x*y"=w476:dbl)
            n165 = expression code="(x/180.0)*pi" "degrees to radians"(0.0) -> (w470:dbl)
            n166 = Negate(x=w476) -> (-x=w479:dbl)
            n167 = call "remote co.vi"("input"=w475) -> ("x*y"=w474:dbl)
            n168 = Re/Im To Polar(2:w474, 3:w479) -> (0:w471:dbl, 1:w481:dbl)
            n169 = Add(x=w471, y=w470) -> (x+y=w469:dbl)
            n170 = call "remote co.vi"("input"=w472) -> ("x*y"=w473:dbl)
            n171 = call "move direction V1.2.vi"("theta"=w469) -> ("out array"=w480:dbl[])  [unwired: 1 in, 1 out]
            n172 = Multiply(x=w480, y=w481) -> (x*y=w483:dbl[])
            n173 = Multiply(x=w473, y=dbl[] [1.0, 1.0, 1.0]) -> (x*y=w482:dbl[])
            n174 = Add(x=w483, y=w482) -> (x+y=w478:dbl[])
            n175 = Select(t=0.9 ("y"), s=w462, f=1.1) -> (s? t:f=w463:dbl)
            n176 = Divide(x=w478, y=w463) -> (x/y=w466:dbl[])
            n177 = Equal?(x=w490, y=7) -> (x = y?=w491:bool)
          }
          frame "reg_catch" {
            # "register catch"
            n178 = Unbundle By Name(w507) -> ("Lx"=w527:i16, "Ly"=w526:i16, "Rx"=w525:i16)
            n179 = To Double Precision Float(number=w527) -> (double precision float=w517:dbl)
            n180 = To Double Precision Float(number=w526) -> (double precision float=w515:dbl)
            n181 = To Double Precision Float(number=w525) -> (double precision float=w512:dbl)
            n182 = call "remote reg catch.vi"("catch? in"=w533, "dir in"=w534, "height in"=w538, "reg"=w528, "dt"=w535, "delay timer in"=w540, "PC in"=w541) -> ("delay timer out"=w537:i32, "PC out"=w530:i32, "height out"=w539:dbl, "dir out"=w536:i32, "catch? out"=w532:bool)
            n183 = call "remote co.vi"("input"=w517) -> ("x*y"=w516:dbl)
            n184 = expression code="(x/180.0)*pi" "degrees to radians"(0.0) -> (w510:dbl)
            n185 = Negate(x=w516) -> (-x=w519:dbl)
            n186 = call "remote co.vi"("input"=w515) -> ("x*y"=w514:dbl)
            n187 = Re/Im To Polar(2:w514, 3:w519) -> (0:w511:dbl, 1:w521:dbl)
            n188 = Add(x=w511, y=w510) -> (x+y=w509:dbl)
            n189 = call "remote co.vi"("input"=w512) -> ("x*y"=w513:dbl)
            n190 = call "move direction V1.2.vi"("theta"=w509) -> ("out array"=w520:dbl[])  [unwired: 1 in, 1 out]
            n191 = Multiply(x=w520, y=w521) -> (x*y=w523:dbl[])
            n192 = Multiply(x=w513, y=dbl[] [1.0, 1.0, 1.0]) -> (x*y=w522:dbl[])
            n193 = Add(x=w523, y=w522) -> (x+y=w518:dbl[])
            n194 = Select(t=0.9 ("y"), s=w503, f=1.1) -> (s? t:f=w502:dbl)
            n195 = Divide(x=w518, y=w502) -> (x/y=w506:dbl[])
            n196 = Equal?(x=w530, y=7) -> (x = y?=w531:bool)
          }
          frame "box_catch" {
            w545 = T9[] [enum."box 3 pre", enum."box 2 pre", enum."box 1 pre", enum."box 3", enum."box 2", enum."box 1"] items=["IDLE", "recycle pre-catch", "recycle catch", "recycle zone", "vision height", "box 1", "box 2", "box 3", "box 1 pre", "box 2 pre", "box 3 pre", "reg 1", "reg 2", "reg 1 pre", "reg 2 pre", "put 1", "put 2", "put 3"] ("height name")
            # "box catch"
            n197 = Index Array(array=w545, index=w542) -> (element=w544:T9)
            n198 = Equal To 0?(x=w550) -> (x = 0?=w549:bool)
            n199 = call "height set.vi"("height name"=w544) -> ("Numeric"=w551:dbl)  [unwired: 10 in]
            n200 = call "raise Height state.vi"("Enum"=enum16{"read", "write"}."read") -> ("read Height"=w547:dbl)  [unwired: 9 in, 1 out]
            n201 = Select(t=w551, s=w549, f=w547) -> (s? t:f=w546:dbl)
          }
        }
        n202 = Select(t="NONE", s=w153, f=w152) -> (s? t:f=w150:string)
      }
      frame True {
        w589 = 0
        n203 = Unbundle By Name(w559) -> ("Up"=w588:bool, "Right"=w587:bool, "Down"=w586:bool)
        n204 = Unbundle By Name(w559) -> ("Down"=w583:bool, "Left"=w582:bool, "Up"=w581:bool, "Right"=w580:bool, "B"=w572:bool)
        n205 = Unbundle By Name(w559) -> ("RT"=w627:i16, "LT"=w629:i16)  [unwired: 1 out]
        n206 = Unbundle By Name(w559) -> ("Lx"=w651:i16, "Ly"=w650:i16, "Rx"=w649:i16)
        n207 = Unbundle By Name(w559) -> ("B"=w567:bool, "RB"=w602:bool, "LB"=w607:bool, "A"=w599:bool)
        n208 = feedback #5(w602) -> (w604:bool)
        n209 = feedback-in #5(w602) -> ()
        n210 = feedback #6(w607) -> (w608:bool)
        n211 = feedback-in #6(w607) -> ()
        n212 = feedback #7(w599) -> (w600:bool)
        n213 = feedback-in #7(w599) -> ()
        n214 = Build Array(w588, w587, w586) -> (w585:bool[])
        n215 = To Double Precision Float(number=w651) -> (double precision float=w640:dbl)
        n216 = To Double Precision Float(number=w650) -> (double precision float=w638:dbl)
        n217 = To Double Precision Float(number=w649) -> (double precision float=w635:dbl)
        n218 = Negate(x=w629) -> (-x=w628:i16)
        n219 = Build Array(w583, w582, w581, w580) -> (w563:bool[])
        n220 = Add(x=w627, y=w628) -> (x+y=w594:i16)
        n221 = Select(t="NONE", s=w572, f=w571) -> (s? t:f=w573:string)
        n222 = feedback-in #8(w563) -> ()
        n223 = feedback #8(w563) -> (w564:bool[])
        n224 = Not(x=w604) -> (.not. x?=w605:bool)
        n225 = Not(x=w608) -> (.not. x?=w609:bool)
        n226 = Not(x=w600) -> (.not. x?=w601:bool)
        n227 = call "remote co.vi"("input"=w640) -> ("x*y"=w639:dbl)
        n228 = Search 1D Array(1D array=w585, element=TRUE) -> ()  [unwired: 1 in, 1 out]
        n229 = expression code="(x/180.0)*pi" "degrees to radians"(0.0) -> (w633:dbl)
        n230 = And(x=w602, y=w605) -> (x .and. y?=w603:bool)
        n231 = And(x=w607, y=w609) -> (x .and. y?=w606:bool)
        n232 = And(x=w599, y=w601) -> (x .and. y?=w598:bool)
        n233 = Negate(x=w639) -> (-x=w642:dbl)
        n234 = call "remote co.vi"("input"=w638) -> ("x*y"=w637:dbl)
        n235 = To Double Precision Float(number=w594) -> (double precision float=w624:dbl)
        n236 = Not(x=w564) -> (.not. x?=w562:bool[])
        n237 = Not(x=w596) -> (.not. x?=w597:bool)
        n238 = And(x=w563, y=w562) -> (x .and. y?=w561:bool[])
        n239 = Select(t=w597, s=w598, f=w596) -> (s? t:f=w595:bool)
        n240 = Re/Im To Polar(2:w637, 3:w642) -> (0:w634:dbl, 1:w644:dbl)
        n241 = Boolean To (0,1)(Boolean=w606) -> (0, 1=w617:i16)
        n242 = Divide(x=w624, y=2.0) -> (x/y=w626:dbl)
        n243 = Add(x=w634, y=w633) -> (x+y=w632:dbl)
        n244 = Boolean To (0,1)(Boolean=w603) -> (0, 1=w616:i16)
        n245 = Negate(x=w617) -> (-x=w615:i16)
        n246 = call "remote co.vi"("input"=w635) -> ("x*y"=w636:dbl)
        n247 = call "remote co.vi"("input"=w626) -> ("x*y"=w619:dbl)
        n248 = Search 1D Array(1D array=w561, element=TRUE) -> (index of element=w578:i32)  [unwired: 1 in]
        n249 = Add(x=w616, y=w615) -> (x+y=w614:i16)
        n250 = Increment(x=w578) -> (x+1=w577:i32)
        n251 = call "move direction V1.2.vi"("theta"=w632) -> ("out array"=w643:dbl[])  [unwired: 1 in, 1 out]
        n252 = Multiply(x=0.001 ("value"), y=w619) -> (x*y=w618:dbl)
        n253 = case shown="\"NONE\", Default" w573 {
          selector: w573 -> [_ w657 w663 w669 w676 w687]
          tunnel: w577 -> [w655 w661 w667 w673 w682 w690]
          tunnel: [w654 w657 w663 w669 w680 w689] -> w576
          tunnel: [FALSE w658 w664 w670 w681 w685] -> w575
          tunnel: [0 w660 w666 w672 w679 w688] -> w574
          frame "NONE", Default {
            n254 = Index Array(array=string[] ["NONE", "reg_catch", "reg_store", "box_catch", "room_put"], index=w655) -> (element=w654:string)
          }
          frame "reg_store" {
            n255 = Index Array(array=i32[] [-1, 2, -1, 0, 1], index=w661) -> (element=w660:i32)
            n256 = Not Equal?(x=w660, y=-1) -> (x != y?=w658:bool)
          }
          frame "room_put" {
            n257 = Index Array(array=i32[] [-1, 2, 3, 0, 1], index=w667) -> (element=w666:i32)
            n258 = Not Equal?(x=w666, y=-1) -> (x != y?=w664:bool)
          }
          frame "reg_catch" {
            n259 = Index Array(array=i32[] [-1, 2, -1, 0, 1], index=w673) -> (element=w672:i32)
            n260 = Not Equal?(x=w672, y=-1) -> (x != y?=w670:bool)
          }
          frame "box_catch" {
            n261 = Index Array(array=i32[] [-1, 2, -2, 0, 1], index=w682) -> (element=w679:i32)
            n262 = Equal?(x=w679, y=-2) -> (x = y?=w677:bool)
            n263 = Select(t="box_catch_", s=w677, f=w676) -> (s? t:f=w680:string)
            n264 = Greater Or Equal?(x=w679, y=0) -> (x >= y?=w681:bool)
          }
          frame "box_catch_" {
            n265 = Index Array(array=i32[] [-1, 5, -2, 3, 4], index=w690) -> (element=w688:i32)
            n266 = Greater Or Equal?(x=w688, y=0) -> (x >= y?=w685:bool)
            n267 = Select(t="box_catch", s=w685, f=w687) -> (s? t:f=w689:string)
          }
        }
        n268 = Add(x=w614, y=w613) -> (x+y=w612:i32)
        n269 = Multiply(x=w643, y=w644) -> (x*y=w647:dbl[])
        n270 = Multiply(x=w636, y=dbl[] [1.0, 1.0, 1.0]) -> (x*y=w646:dbl[])
        n271 = Add(x=w647, y=w646) -> (x+y=w641:dbl[])
        n272 = Add(x=w618, y=w623) -> (x+y=w560:dbl)
        n273 = In Range and Coerce(upper limit=1, x=w612, lower limit=-1) -> (coerced(x)=w593:i32)  [unwired: 1 out]
        n274 = Select(t=0.9 ("y"), s=w557, f=1.1) -> (s? t:f=w558:dbl)
        n275 = Divide(x=w641, y=w558) -> (x/y=w630:dbl[])
        n276 = In Range and Coerce(upper limit=28.3, x=w560, lower limit=0.0) -> (coerced(x)=w568:dbl)  [unwired: 1 out]
        n277 = call "raise Height state.vi"("Enum"=enum16{"read", "write"}."read") -> ("read Height"=w565:dbl)  [unwired: 9 in, 1 out]
        n278 = Select(t=w565, s=w567, f=w568) -> (s? t:f=w569:dbl)
        n279 = Select(t=FALSE, s=w575, f=w591) -> (s? t:f=w592:bool)
      }
    }
    n280 = Bundle By Name(cluster=T8 {"Motor speed"=[], "height"=0.0, "dir"=0, "catch?"=FALSE} ("write"), "Motor speed"=w137, "height"=w129, "dir"=w128, "catch?"=w130) -> (w135:T8)
    n281 = call "remote-reg.vi"("Enum"=enum16{"read", "write"}."write", "write"=w135) -> ()  [unwired: 9 in, 1 out]
    n282 = node-c288() -> ()  [unwired: 1 in, 1 out]
  }
  n283 = node-c288(w26) -> ()  [unwired: 1 out]
  n284 = call "3motor.vi"("error in (no error)"=w21, "Reset"=TRUE) -> ()  [unwired: 8 in, 2 out]
  n285 = node-c288(w31) -> ()  [unwired: 1 out]
  n286 = call <userlib>:"f710_close.vi"("error in (no error)"=w28, "VISA Refnum in"=w29) -> ("error out"=→"error out":errorcluster)  [unwired: 9 in]
